vi "Create exchange (SubVI).vi"(0 "Connection in":refnum<class "Connection.lvclass">, 1 "exchange name":u16(ring) items=["requests", "alerts"], 2 "error in (no error)":errorcluster) -> (3 "Connection out":refnum<class "Connection.lvclass">, 4 "Exchange.lvclass":refnum<class "Exchange.lvclass">, 5 "Channel out":refnum<class "Channel.lvclass">, 6 "error out":errorcluster)   [LabVIEW 2016]
uses:
  <vilib>/Distrio/LabbitMQ/Connection/Connection.lvclass
  <vilib>/Distrio/LabbitMQ/Exchange/Exchange.lvclass
  <vilib>/Distrio/LabbitMQ/Channel/Channel.lvclass
  <vilib>/Distrio/LabbitMQ/Channel/exchange_type_enum.ctl
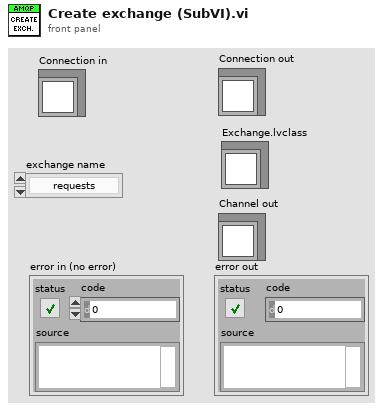
[diagram p1: front panel]
types:
  T1 = typedef "Channel.lvclass/exchange_type_enum.ctl" = enum16{"direct", "topic", "fanout", "headers"}
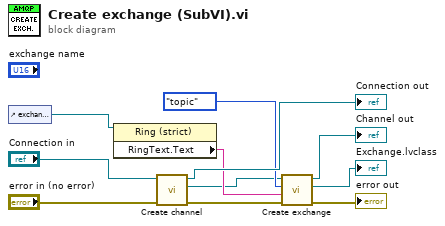
[diagram p0: block diagram]
diagram:
  n1 = control-ref of="exchange name"() -> (w2:refnum<vi>)
  n2 = property on="Property Node" class="Ring (strict)"(reference=w2) -> ("RingText.Text"=w10:string)  [unwired: 1 in, 2 out]
  n3 = call <vilib>:"Create channel.vi"("error in (no error)"="error in (no error)", "Connection in"="Connection in") -> ("error out"=w6:errorcluster, "channel"=w5:refnum<class "Channel.lvclass">, "Connection out"=→"Connection out":refnum<class "Connection.lvclass">)  [unwired: 7 in]
  n4 = call <vilib>:"Create exchange.vi"("error in (no error)"=w6, "exchange name"=w10, "exchange type"=exchange_type_enum."topic", "Channel in"=w5) -> ("error out"=→"error out":errorcluster, "Exchange.lvclass"=→"Exchange.lvclass":refnum<class "Exchange.lvclass">, "Channel out"=→"Channel out":refnum<class "Channel.lvclass">)  [unwired: 5 in]
